vi "Ocelot.vi"(9 "RCW (X2)":dbl(slide) scale=-1.0..1.0, 10 "FWD (Y)":dbl(slide) scale=-1.0..1.0, 11 "STR (X)":dbl(slide) scale=-1.0..1.0) -> (0 "FRD":dbl(slide) scale=-1.0..1.0, 1 "FLD":dbl(slide) scale=-1.0..1.0, 2 "BRS":dbl(knob) scale=0.0..360.0, 3 "BLS":dbl(knob) scale=0.0..360.0, 4 "BLD":dbl(slide) scale=-1.0..1.0, 5 "FRS":dbl(knob) scale=0.0..360.0, 6 "BRD":dbl(slide) scale=-1.0..1.0, 7 "FLS":dbl(knob) scale=0.0..360.0)   [LabVIEW 2012]
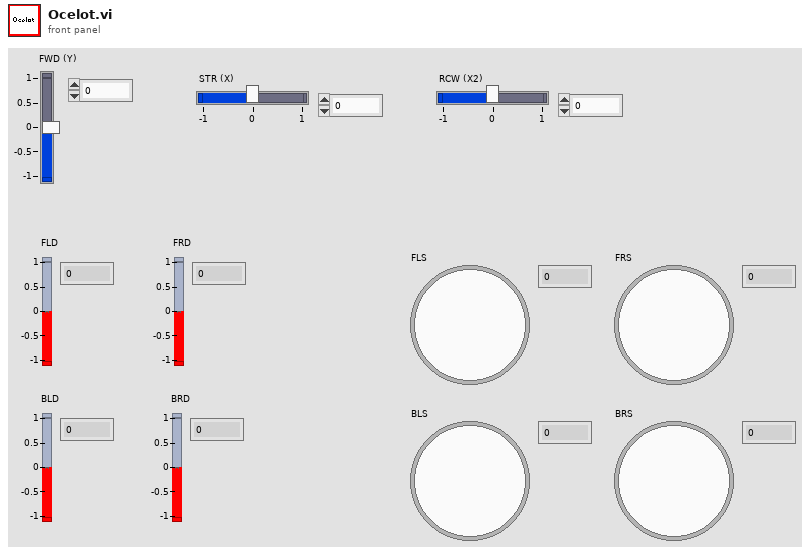
[diagram p1: front panel]
types:
  T1 = cluster{"WD1":dbl, "WD2":dbl, "WD3":dbl, "WD4":dbl}
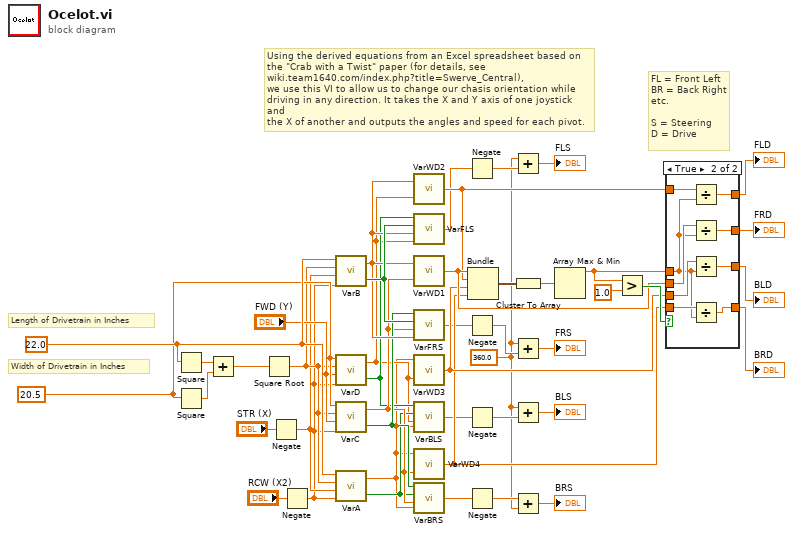
[diagram p0: block diagram]
diagram:
  w11 = 360.0
  w40 = 20.5 ("W")
  w42 = 22.0 ("L")
  # "FL = Front Left\nBR = Back Right\netc.\n\nS = Steering\nD = Drive"
  # "Using the derived equations from an Excel spreadsheet based on\nthe \"Crab with a Twist\" paper (for details, see\nwiki.team1640.com/index.php?title=Swerve_Central),\nwe use this VI to allow us to change our chasis orientation while\ndriving in any direction. It takes the X and Y axis of one joystick and\nthe X of another and outputs the angles and speed for each pivot."
  # "Length of Drivetrain in Inches"
  # "Width of Drivetrain in Inches"
  n1 = Square(x=w42) -> (x^2=w45:dbl)
  n2 = Square(x=w40) -> (x^2=w44:dbl)
  n3 = Add(x=w45, y=w44) -> (x+y=w43:dbl)
  n4 = Square Root(x=w43) -> (sqrt(x)=w37:dbl)
  n5 = Negate(x="STR (X)") -> (-x=w2:dbl)
  n6 = Negate(x="RCW (X2)") -> (-x=w1:dbl)
  n7 = call "VarB.vi"("RCW (X2)"=w1, "STR (X)"=w2, "R"=w37, "L"=w42) -> ("B = 0?"=w27:bool, "B"=w26:dbl)
  n8 = call "VarD.vi"("RCW (X2)"=w1, "FWD (Y)"="FWD (Y)", "R"=w37, "W"=w40) -> ("x = 0?"=w23:bool, "D"=w21:dbl)
  n9 = call "VarC.vi"("RCW (X2)"=w1, "FWD (Y)"="FWD (Y)", "R"=w37, "W"=w40) -> ("C = 0?"=w25:bool, "C"=w24:dbl)
  n10 = call "VarA.vi"("RCW (X2)"=w1, "STR (X)"=w2, "R"=w37, "L"=w42) -> ("A = 0?"=w22:bool, "A"=w20:dbl)
  n11 = call "VarWD2.vi"("D"=w21, "B"=w26) -> ("WD2"=w31:dbl)
  n12 = call "VarFLS.vi"("D"=w21, "B"=w26, "B=0"=w27, "D=0"=w23) -> ("FLS"=w4:dbl)
  n13 = call "VarWD1.vi"("C"=w24, "B"=w26) -> ("WD1"=w32:dbl)
  n14 = call "VarFRS.vi"("B"=w26, "C"=w24, "B=0"=w27, "C=0"=w25) -> ("FRS"=w6:dbl)
  n15 = call "VarWD3.vi"("D"=w21, "A"=w20) -> ("WD3"=w30:dbl)
  n16 = call "VarBLS.vi"("A"=w20, "D"=w21, "A=0"=w22, "D=0"=w23) -> ("BLS"=w8:dbl)
  n17 = call "VarWD4.vi"("C"=w24, "A"=w20) -> ("WD4"=w29:dbl)
  n18 = call "VarBRS.vi"("A"=w20, "C"=w24, "A=0"=w22, "C=0"=w25) -> ("BRS"=w10:dbl)
  n19 = Negate(x=w4) -> (-x=w15:dbl)
  n20 = Negate(x=w6) -> (-x=w14:dbl)
  n21 = Negate(x=w8) -> (-x=w13:dbl)
  n22 = Negate(x=w10) -> (-x=w12:dbl)
  n23 = Bundle("WD1"=w32, "WD2"=w31, "WD3"=w30, "WD4"=w29) -> (w35:T1)  [unwired: 1 in]
  n24 = Add(x=w11, y=w15) -> (x+y=→"FLS":dbl)
  n25 = Cluster To Array(cluster=w35) -> (array=w36:dbl[])
  n26 = Add(x=w11, y=w14) -> (x+y=→"FRS":dbl)
  n27 = Add(x=w11, y=w13) -> (x+y=→"BLS":dbl)
  n28 = Add(x=w12, y=w11) -> (x+y=→"BRS":dbl)
  n29 = Array Max & Min(array=w36) -> (max value=w28:dbl)  [unwired: 3 out]
  n30 = Greater?(x=w28, y=1.0) -> (0:w33:bool)
  n31 = case shown="True" w33 {
    tunnel: [w49 w54] -> w18
    tunnel: w32 -> [w49 w57]
    tunnel: w31 -> [w48 w58]
    tunnel: w30 -> [w47 w55]
    tunnel: w29 -> [w46 w56]
    tunnel: [w48 w53] -> w19
    tunnel: [w47 w52] -> w17
    tunnel: [w46 w50] -> w16
    tunnel: w28 -> [_ w51]
    frame False {
    }
    frame True {
      n32 = Divide(x=w58, y=w51) -> (x/y=w53:dbl)
      n33 = Divide(x=w57, y=w51) -> (x/y=w54:dbl)
      n34 = Divide(x=w55, y=w51) -> (x/y=w52:dbl)
      n35 = Divide(x=w56, y=w51) -> (x/y=w50:dbl)
    }
  }
  "FRD" <- w18
  "FLD" <- w19
  "BLD" <- w17
  "BRD" <- w16
